vi "bit2char.vi"(10 "input bit stream":i8[](array[numeric])) -> (2 "数据字符串 2":string)   [LabVIEW 2010]
panel:
  out "数组 2":i8[](array[numeric])
  out "大小":i32
  out "输出数组":i8[][](array[numeric])
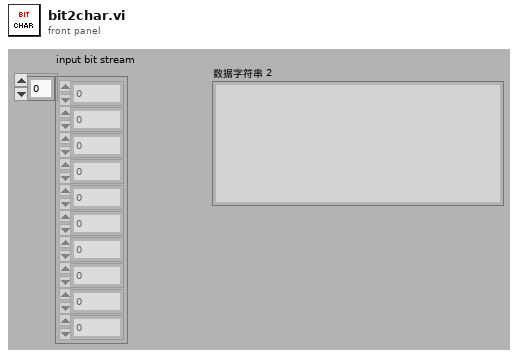
[diagram p1: front panel]
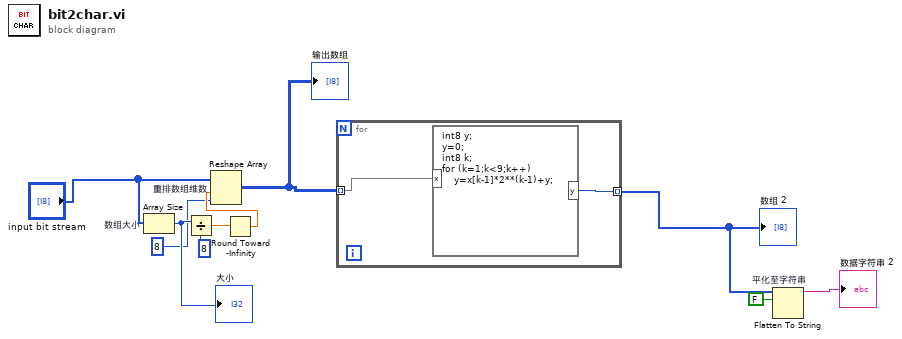
[diagram p0: block diagram]
diagram:
  n1 = Array Size "数组大小"(array="input bit stream") -> (size(s)=w10:i32)
  "大小" <- w10
  n2 = Divide(x=w10, y=8) -> (x/y=w8:dbl)
  n3 = Round Toward -Infinity(1:w8) -> (0:w7:dbl)
  n4 = Reshape Array "重排数组维数"("input bit stream", w7, 8 ("维数大小")) -> (w5:i8[][])
  "输出数组" <- w5
  n5 = for {
    tunnel: w5 -> [w12] mode=indexing
    tunnel: [w11] -> w1 mode=indexing
    n6 = formula code="int8 y;\ny=0;\nint8 k;\nfor (k=1;k<9;k++)\n    y=x[k-1]*2**(k-1)+y;"("x"=w12) -> ("y"=w11:i8)
  }
  "数组 2" <- w1
  n7 = Flatten To String "平化至字符串"(anything=w1, prepend array or string size? (T)=FALSE ("预置数组或字符串大小？(T)")) -> (data string=→"数据字符串 2":string)  [unwired: 2 in, 2 out]
